vi "CMD_ATAN2.vi"(8 "error in (no error)":errorcluster, 10 "Arguments":string[](array[string]), 11 "gScript Interpreter in":refnum<class "gScript Interpreter.lvclass">) -> (0 "error out":errorcluster, 3 "gScript Interpreter out":refnum<class "gScript Interpreter.lvclass">)   [LabVIEW 2017, in "gScript Interpreter.lvclass"]
uses:
  gScript Interpreter.lvclass
  Type Definitions/Memory Cell.ctl
  Type Definitions/Memory Cell Type Enum.ctl
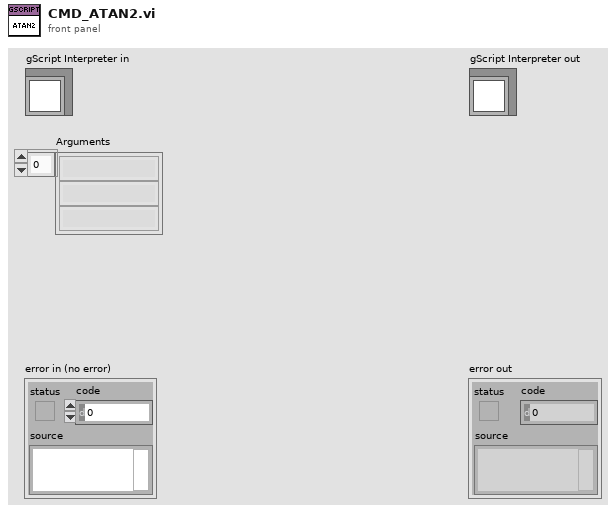
[diagram p1: front panel]
types:
  T1 = typedef "Memory Cell Type Enum.ctl" = enum16{"integer", "float", "vector", "rotation"}
  T2 = typedef "Memory Cell.ctl" = cluster{"type":T1, "x":dbl, "y":dbl, "z":dbl, "w":dbl}
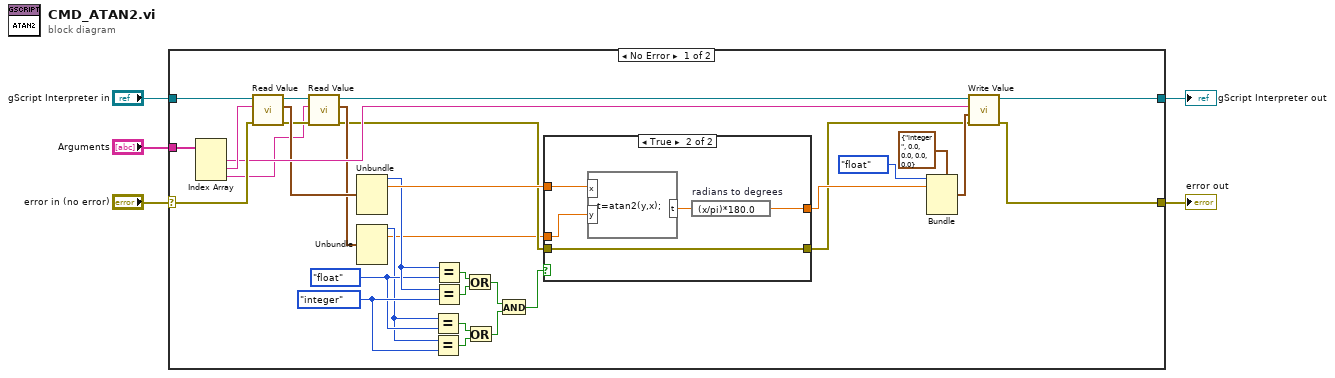
[diagram p0: block diagram]
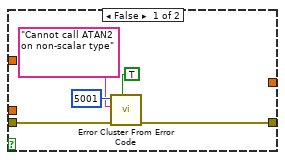
[diagram p2: hidden frame]
diagram:
  n1 = case shown="No Error" "error in (no error)" {
    selector: "error in (no error)" -> [w35 w49]
    tunnel: [w28 w49] -> w4
    tunnel: [w29 w48] -> w2
    tunnel: "gScript Interpreter in" -> [w36 w48]
    tunnel: "Arguments" -> [w37 _]
    frame No Error {
      w16 = Memory_Cell_Type_Enum."integer" ("type")
      w15 = Memory_Cell_Type_Enum."float" ("type")
      n2 = Index Array(array=w37) -> (element #1=w33:string, element #2=w34:string, element #3=w21:string)  [unwired: 3 in]
      n3 = call-dynamic "Read Value.vi"("error in (no error)"=w35, "String in"=w34, "gScript Interpreter in"=w36) -> ("error out"=w22:errorcluster, "Memory Cell"=w32:T2, "gScript Interpreter out"=w23:refnum<class "gScript Interpreter.lvclass">)  [unwired: 6 in]
      n4 = call-dynamic "Read Value.vi"("error in (no error)"=w22, "String in"=w21, "gScript Interpreter in"=w23) -> ("error out"=w18:errorcluster, "Memory Cell"=w20:T2, "gScript Interpreter out"=w19:refnum<class "gScript Interpreter.lvclass">)  [unwired: 6 in]
      n5 = Unbundle(w32) -> ("type"=w17:T1, "x"=w27:dbl)  [unwired: 3 out]
      n6 = Unbundle(w20) -> ("type"=w14:T1, "x"=w6:dbl)  [unwired: 3 out]
      n7 = Equal?(x=w14, y=w15) -> (x = y?=w11:bool)
      n8 = Equal?(x=w14, y=w16) -> (x = y?=w10:bool)
      n9 = Equal?(x=w17, y=w15) -> (x = y?=w12:bool)
      n10 = Equal?(x=w17, y=w16) -> (x = y?=w13:bool)
      n11 = Or(x=w12, y=w13) -> (x .or. y?=w9:bool)
      n12 = Or(x=w11, y=w10) -> (x .or. y?=w8:bool)
      n13 = And(x=w9, y=w8) -> (x .and. y?=w7:bool)
      n14 = case shown="True" w7 {
        tunnel: w27 -> [_ w46]
        tunnel: [_ w43] -> w26
        tunnel: w18 -> [w38 w47]
        tunnel: [w42 w47] -> w24
        tunnel: w6 -> [_ w45]
        frame False {
          n15 = call <vilib>:"Error Cluster From Error Code.vi"("show call chain? (False)"=TRUE, "error in (no error)"=w38, "error message (\"\")"="Cannot call ATAN2 on non-scalar type" ("error message (\"\")"), "error code (0)"=5001) -> ("error out"=w42:errorcluster)  [unwired: 5 in]
        }
        frame True {
          n16 = formula code="t=atan2(y,x);"("x"=w46, "y"=w45) -> ("t"=w44:dbl)
          n17 = expression code="(x/pi)*180.0" "radians to degrees"(w44) -> (w43:dbl)
        }
      }
      n18 = Bundle(cluster=T2 {"type"=enum."integer", "x"=0.0, "y"=0.0, "z"=0.0, "w"=0.0} ("Memory Cell"), "type"=Memory_Cell_Type_Enum."float", "x"=w26) -> (w30:T2)  [unwired: 3 in]
      n19 = call-dynamic "Write Value.vi"("error in (no error)"=w24, "Value"=w30, "Address"=w33, "gScript Interpreter in"=w19) -> ("error out"=w28:errorcluster, "gScript Interpreter out"=w29:refnum<class "gScript Interpreter.lvclass">)  [unwired: 6 in]
    }
    frame Error {
    }
  }
  "error out" <- w4
  "gScript Interpreter out" <- w2
